vi "Shortest Distance.vi"(10 "target":dbl(knob) scale=0.0..360.0, 11 "current":dbl(knob) scale=0.0..360.0) -> (0 "flipping?":bool, 3 "angle to rotate":dbl)   [LabVIEW 2014]
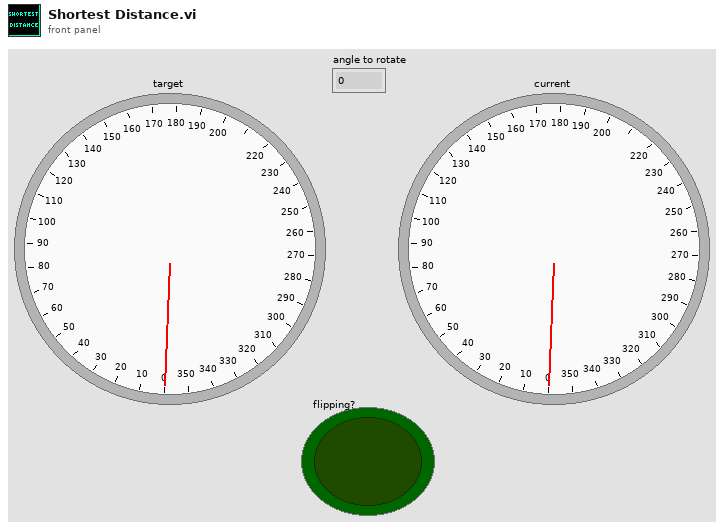
[diagram p1: front panel]
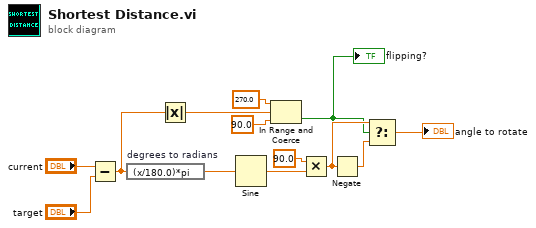
[diagram p0: block diagram]
diagram:
  n1 = Subtract(x="current", y="target") -> (x-y=w8:dbl)
  n2 = expression code="(x/180.0)*pi" "degrees to radians"(w8) -> (w11:dbl)
  n3 = Absolute Value(x=w8) -> (abs(x)=w7:dbl)
  n4 = Sine(x=w11) -> (sin(x)=w9:dbl)
  n5 = In Range and Coerce(upper limit=270.0, x=w7, lower limit=90.0) -> (In Range?=w1:bool)  [unwired: 1 out]
  "flipping?" <- w1
  n6 = Multiply(x=90.0, y=w9) -> (x*y=w4:dbl)
  n7 = Negate(x=w4) -> (-x=w3:dbl)
  n8 = Select(t=w4, s=w1, f=w3) -> (s? t:f=→"angle to rotate":dbl)
